vi "Read Measurement.vi"   [LabVIEW 2021, in "Yokogawa WT1800 Series.lvlib"]
doc: "Queries the waveform measurement value.\n\nNote:\n(1) If the measurement is not possible, \"NAN (Not A Number)\" is returned."
uses:
  <instrlib>/Yokogawa WT1800 Series/Yokogawa WT1800 Series.lvlib
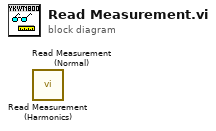
[diagram p0: block diagram]
diagram:
  n1 = call <instrlib>:"Read Measurement (Harmonics).vi"() -> ()  [unwired: 8 in, 4 out]
  n2 = call <instrlib>:"Read Measurement (Normal).vi"() -> ()  [unwired: 8 in, 4 out]
